vi "App - FileSync Example.vi"() -> ()   [LabVIEW 2020]
uses:
  FTP/FTPProtocol/FTPProtocol.lvclass
  C:/Users/liyao/Desktop/JKISM-FileSync/Base/Protocol/Protocol.lvclass
  Base/FileSync -- Base.lvlib
  <userlib>/_NEVSTOP/JKI State Machine ++/JKI-State-Machine-Plus.lvlib
panel:
  in  "Hide FP":bool
  in  "Show FP":bool
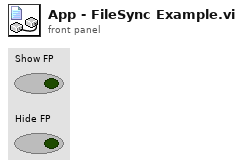
[diagram p1: front panel]
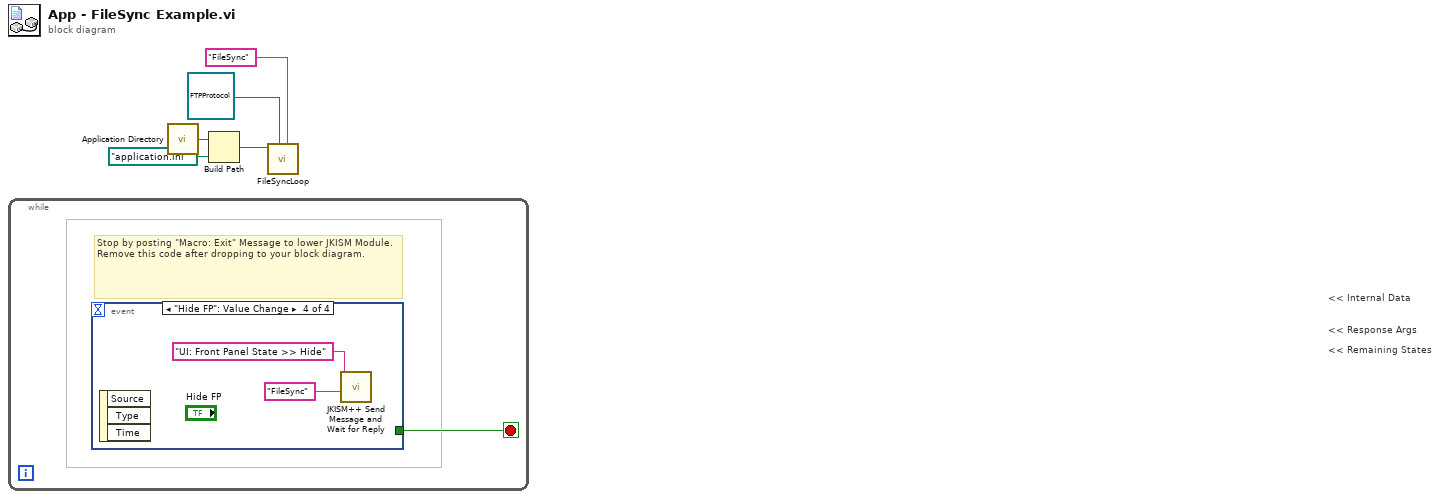
[diagram p0: block diagram]
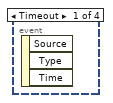
[diagram p2: hidden frame]
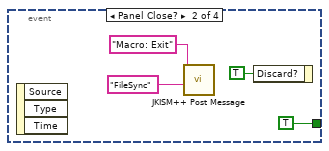
[diagram p3: hidden frame]
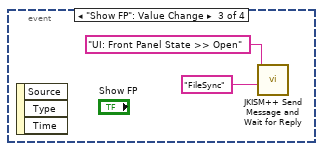
[diagram p4: hidden frame]
diagram:
  # "<< Internal Data"
  # "<< Response Args"
  # "<< Remaining States"
  n1 = while {
    stop <- w6 stop-if-true
    # "Stop by posting \"Macro: Exit\" Message to lower JKISM Module. Remove this code after dropping to your block diagram."
    n2 = event shown="[3] \"Hide FP\": Value Change" {
      selector: _ -> [_ _ _ _]
      dyn-events: _ -> [_ _ _ _]
      timeout: _ -> [_ _ _ _]
      tunnel: [_ TRUE _ _] -> w6
      event Timeout {
        n3 = event-data() -> ()  [unwired: 1 in, 3 out]
      }
      event Panel Close? {
        n4 = event-data() -> ()  [unwired: 1 in, 3 out]
        n5 = call <userlib>:"JKISM++ Post Message.vi"("Dest Module"="FileSync" ("Name(FileSync)"), "States"="Macro: Exit") -> ()  [unwired: 9 in, 1 out]
        n6 = event-data("Discard?"=TRUE) -> ()  [unwired: 1 in, 1 out]
      }
      event "Show FP": Value Change {
        n7 = event-data() -> ()  [unwired: 1 in, 3 out]
        n8 = call <userlib>:"JKISM++ Send Message and Wait for Reply.vi"("Dest Module"="FileSync" ("Name(FileSync)"), "States"="UI: Front Panel State >> Open") -> ()  [unwired: 8 in, 2 out]
      }
      event "Hide FP": Value Change {
        n9 = event-data() -> ()  [unwired: 1 in, 3 out]
        n10 = call <userlib>:"JKISM++ Send Message and Wait for Reply.vi"("Dest Module"="FileSync" ("Name(FileSync)"), "States"="UI: Front Panel State >> Hide") -> ()  [unwired: 8 in, 2 out]
      }
    }
  }
  n11 = call <vilib>:"Application Directory.vi"() -> ("Application Directory"=w3:path)
  n12 = Build Path(base path=w3, name or relative path=path "application.ini" ("Path")) -> (appended path=w1:path)
  n13 = call "FileSyncLoop.vi"("Name(FileSync)"="FileSync", "Protocol.lvclass"=refnum<class "FTPProtocol.lvclass"> refnum ("FTPProtocol"), "IniConfigFilePath"=w1) -> ()  [unwired: 8 in, 1 out]
